vi "Configure Measurement (Power Meter - Average).vi"(0 "VISA resource name":refnum<visa-resource-name>, 1 "Enable Step Detect (F: Disable)":bool, 5 "Auto Average Count (F: Disable)":bool, 9 "Average Count Number (2)":dbl=2.0, 11 "error in (no error)":errorcluster) -> (4 "VISA resource name out":refnum<visa-resource-name>, 15 "error out":errorcluster)   [LabVIEW 2022 SP3, in "Agilent N934X Series.lvlib"]
doc: "Configures the cable setting of Power Meter Average.\n\nNotes:\n(1) Option PWM or PWP is required to enable this function. Option PWM supports Keysight (Agilent) U2000 series USB average power sensor, and Option PWP supports Keysight (Agilent) U2020 X series peak power sensor.\n\n(2) This VI is only applicable for N9321C, N9322C, N9323C, N9324C models"
uses:
  <instrlib>/Agilent N934X Series/Agilent N934X Series.lvlib
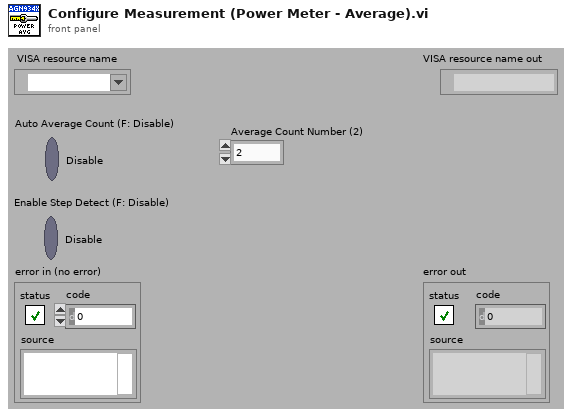
[diagram p1: front panel]
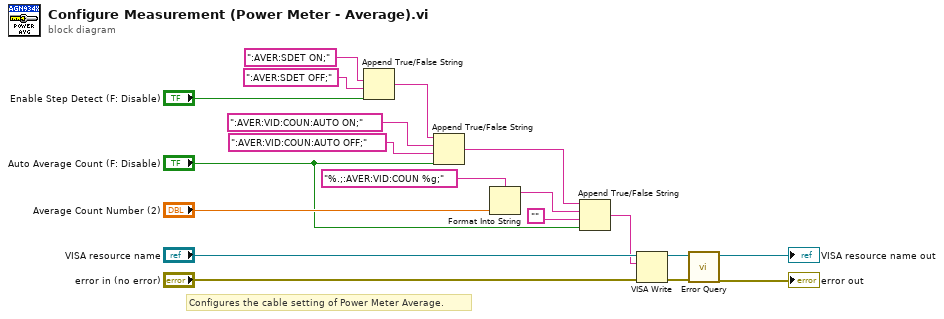
[diagram p0: block diagram]
diagram:
  # "Configures the cable setting of Power Meter Average."
  n1 = Append True/False String(1:"Enable Step Detect (F: Disable)", 2:":AVER:SDET OFF;", 3:":AVER:SDET ON;") -> (0:w6:string)  [unwired: 1 in]
  n2 = Append True/False String(1:"Auto Average Count (F: Disable)", 2:":AVER:VID:COUN:AUTO OFF;", 3:":AVER:VID:COUN:AUTO ON;", 4:w6) -> (0:w4:string)
  n3 = Format Into String(format string="%.;:AVER:VID:COUN %g;", "Average Count Number (2)") -> (resulting string=w5:string)  [unwired: 2 in, 1 out]
  n4 = Append True/False String(1:"Auto Average Count (F: Disable)", 2:"", 3:w5, 4:w4) -> (0:w1:string)
  n5 = VISA Write(VISA resource name="VISA resource name", write buffer=w1, error in (no error)="error in (no error)") -> (VISA resource name out=w10:refnum<visa-resource-name>, error out=w9:errorcluster)  [unwired: 1 out]
  n6 = call <instrlib>:"Error Query.vi"("error in (no error)"=w9, "VISA resource name"=w10) -> ("error out"=→"error out":errorcluster, "VISA resource name out"=→"VISA resource name out":refnum<visa-resource-name>)  [unwired: 6 in, 2 out]
